vi "Write Index.vi"(10 "Index":i32, 11 "(Index_Pointer) In":refnum<class "Absolute_Pointer.lvclass">) -> (3 "(Index_Pointer) Out":refnum<class "Absolute_Pointer.lvclass">)   [LabVIEW 2025, in "Absolute_Pointer.lvclass"]
uses:
  Absolute_Pointer.lvclass
  Absolute_Pointer.lvclass/Absolute_Pointer.ctl
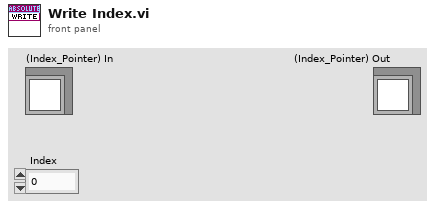
[diagram p1: front panel]
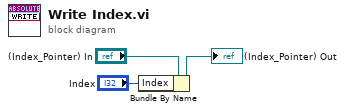
[diagram p0: block diagram]
diagram:
  n1 = Bundle By Name(cluster="(Index_Pointer) In", "Index"="Index") -> (→"(Index_Pointer) Out":refnum<class "Absolute_Pointer.lvclass">)
